vi "Read TCP Data.vi"(8 "error in (no error)":errorcluster) -> (3 "TCP Data":bool)   [LabVIEW 2020]
uses:
  Type Definitions/Terminal Data Source Selector.ctl
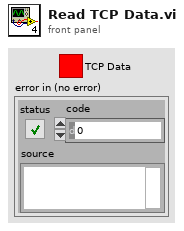
[diagram p1: front panel]
types:
  T1 = typedef "Terminal Data Source Selector.ctl" = enum32{"TCP", "UDP", "Network Stream", "USB", "Multicast"}
  T2 = typedef "PC Network Settings.ctl" = cluster{"TCP/IP Address":string, "TCP/IP Port":u16, "UDP/IP Address":string, "UDP/IP Port":u16, "USB Address":string, "USB Port":u16, "NS Reader Name":string, "NS Writer URL":string}
  T3 = typedef "Data Frame.ctl" = cluster{"Frame Header":T4, "Payload":string, "CRC":u32}
  T4 = typedef "Data Frame Header.ctl" = cluster{"Sync":u32, "Time":dbl, "Nanosecond Counter":i64, "Payload Class":T5, "Payload ID":u16, "Counter":u32, "Options":u32, "Source":i32, "Destination":i32}
  T5 = typedef "Payload Class.ctl" = enum16{"System State", "Parameters", "Metadata", "Software Monitor", "Data", "Commands"}
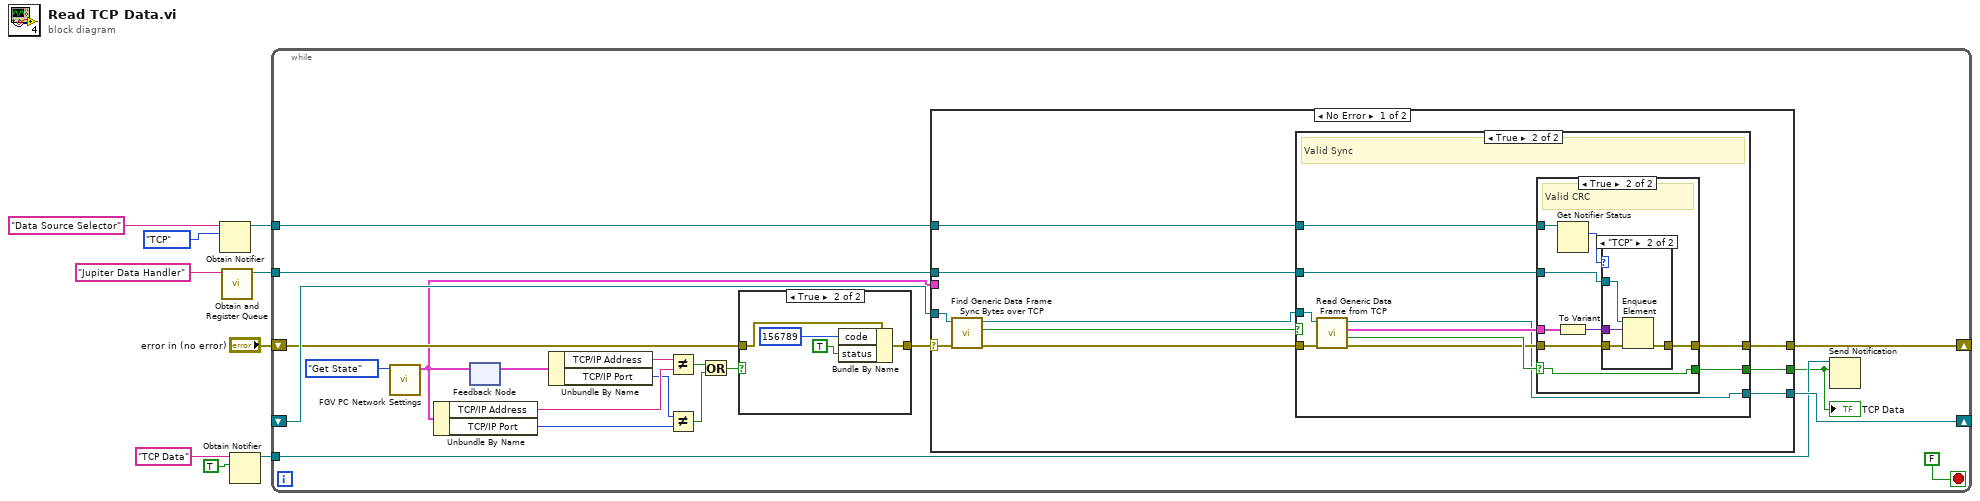
[diagram p0: block diagram]
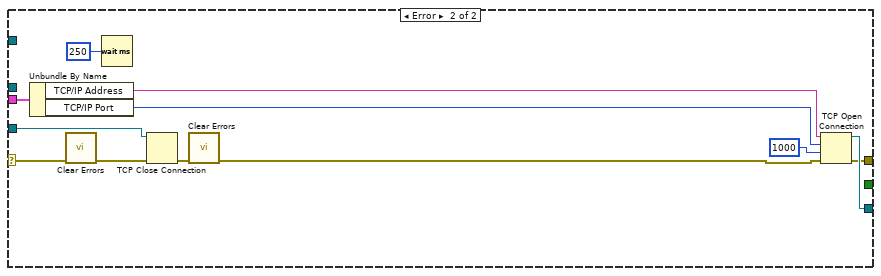
[diagram p6: hidden frame]
diagram:
  n1 = Obtain Notifier(name (unnamed)="Data Source Selector", notification data type=Terminal_Data_Source_Selector."TCP" ("Data Source Selector")) -> (notifier out=w6:refnum<notifier>)  [unwired: 2 in, 2 out]
  n2 = call "Obtain and Register Queue.vi"("name (unnamed)"="Jupiter Data Handler") -> ("Queue Out"=w4:refnum<queue>)  [unwired: 7 in, 3 out]
  n3 = Obtain Notifier(name (unnamed)="TCP Data", notification data type=TRUE) -> (notifier out=w9:refnum<notifier>)  [unwired: 2 in, 2 out]
  n4 = while {
    shift-right: [w29] -> _
    shift-left: "error in (no error)" -> [w19]
    shift-right: [w28] -> _
    shift-left: _ -> [w27]
    tunnel: w4 -> [w25]
    tunnel: w6 -> [w24]
    tunnel: w9 -> [w23]
    stop <- FALSE stop-if-true
    n5 = call "FGV PC Network Settings.vi"("Function"=enum16{"Initialize", "Set State", "Get State"}."Get State") -> ("PC Network Settings Out"=w18:T2)  [unwired: 9 in, 1 out]
    n6 = Unbundle By Name(w18) -> ("TCP/IP Address"=w15:string, "TCP/IP Port"=w13:u16)
    n7 = feedback #1() -> (w17:T2)  [unwired: 1 in]
    n8 = feedback-in #1(w18) -> ()
    n9 = Unbundle By Name(w17) -> ("TCP/IP Address"=w16:string, "TCP/IP Port"=w14:u16)
    n10 = Not Equal?(x=w16, y=w15) -> (x != y?=w11:bool)
    n11 = Not Equal?(x=w14, y=w13) -> (x != y?=w12:bool)
    n12 = Or(x=w11, y=w12) -> (x .or. y?=w10:bool)
    n13 = case shown="True" w10 {
      tunnel: w19 -> [w30 w34]
      tunnel: [w30 w33] -> w20
      frame False {
      }
      frame True {
        n14 = Bundle By Name(cluster=w34, "code"=156789, "status"=TRUE) -> (w33:errorcluster)
      }
    }
    n15 = case shown="No Error" w20 {
      selector: w20 -> [w44 w82]
      tunnel: [w39 w75] -> w29
      tunnel: [w41 w77] -> w28
      tunnel: w27 -> [w43 w78]
      tunnel: w25 -> [w37 _]
      tunnel: [w36 _] -> w22
      tunnel: w24 -> [w35 _]
      tunnel: w18 -> [_ w71]
      frame No Error {
        n16 = call "Find Generic Data Frame Sync Bytes over TCP.vi"("error in (no error)"=w44, "TCP Network Connection in"=w43) -> ("error out"=w40:errorcluster, "Valid Sync"=w38:bool, "TCP Network Connection out"=w42:refnum<k5>)  [unwired: 7 in]
        n17 = case shown="True" w38 {
          tunnel: w42 -> [w46 w56]
          tunnel: [w46 w47] -> w41
          tunnel: w40 -> [w45 w55]
          tunnel: [w45 w50] -> w39
          tunnel: w37 -> [_ w52]
          tunnel: [_ w49] -> w36
          tunnel: w35 -> [_ w48]
          frame False {
            # "Invalid Sync"
          }
          frame True {
            # "Valid Sync"
            n18 = call "Read Generic Data Frame from TCP.vi"("error in (no error)"=w55, "TCP Network Connection in"=w56) -> ("error out"=w51:errorcluster, "Valid CRC"=w53:bool, "Frame Received"=w54:T3, "TCP Network Connection out"=w47:refnum<k5>)  [unwired: 6 in]
            n19 = case shown="True" w53 {
              selector: w53 -> [_ w60]
              tunnel: w54 -> [_ w61]
              tunnel: w52 -> [_ w65]
              tunnel: w51 -> [w57 w64]
              tunnel: [w57 w63] -> w50
              tunnel: [_ w60] -> w49
              tunnel: w48 -> [_ w58]
              frame False {
                # "Invalid CRC"
              }
              frame True {
                # "Valid CRC"
                n20 = Get Notifier Status(notifier=w58) -> (current notification=w59:T1)  [unwired: 1 in, 4 out]
                n21 = To Variant(anything=w61) -> (Variant=w62:variant)
                n22 = case shown="\"TCP\"" w59 {
                  tunnel: w65 -> [_ w70]
                  tunnel: w64 -> [w66 w69]
                  tunnel: [w66 w68] -> w63
                  tunnel: w62 -> [_ w67]
                  frame Default {
                  }
                  frame "TCP" {
                    n23 = Enqueue Element(queue=w70, element=w67, error in (no error)=w69) -> (error out=w68:errorcluster)  [unwired: 1 in, 2 out]
                  }
                }
              }
            }
          }
        }
      }
      frame Error {
        n24 = Unbundle By Name(w71) -> ("TCP/IP Address"=w73:string, "TCP/IP Port"=w72:u16)
        n25 = call <vilib>:"Clear Errors.vi"("error in (no error)"=w82) -> ("error out"=w80:errorcluster)  [unwired: 5 in, 1 out]
        n26 = Wait (ms)(milliseconds to wait=u32 250) -> ()  [unwired: 1 out]
        n27 = TCP Close Connection(connection ID=w78, error in (no error)=w80) -> (error out=w79:errorcluster)  [unwired: 1 in, 1 out]
        n28 = call <vilib>:"Clear Errors.vi"("error in (no error)"=w79) -> ("error out"=w76:errorcluster)  [unwired: 5 in, 1 out]
        n29 = TCP Open Connection(address=w73, remote port or service name=w72, timeout ms (60000)=1000 ("timeout ms (wait forever: -1)"), error in (no error)=w76) -> (connection ID=w77:refnum<k5>, error out=w75:errorcluster)  [unwired: 1 in]
      }
    }
    "TCP Data" <- w22
    n30 = Send Notification(notification=w22, notifier=w23) -> ()  [unwired: 1 in, 2 out]
  }
